vi "FPGA_brightfield_control.vi"() -> ()   [LabVIEW 2015]
uses:
  <vilib>/rvi/Emulation/niFpgaGetClockAttributes.vi
  <vilib>/rvi/Emulation/niFpgaSctlEmulationGetInTimedLoop.vi
  <vilib>/rvi/Emulation/niFpgaEmulationReportErrorSimple.vi
  <vilib>/rvi/Emulation/niFpgaProcessEmulError.vi
  <vilib>/rvi/eio/common/nirviEmuTemplateMethod_errors.vi
  <vilib>/rvi/Emulation/niFpgaCriticalErrorInLSC.vi
  <vilib>/eio/EIONode/EIONode.xnode
panel:
  in  "Period":u32
  in  "Triggers length (µs)":u32
  in  "stop":bool
  in  "Intensity":sgl
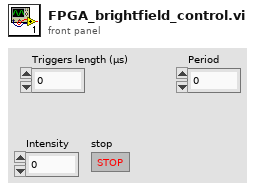
[diagram p1: front panel]
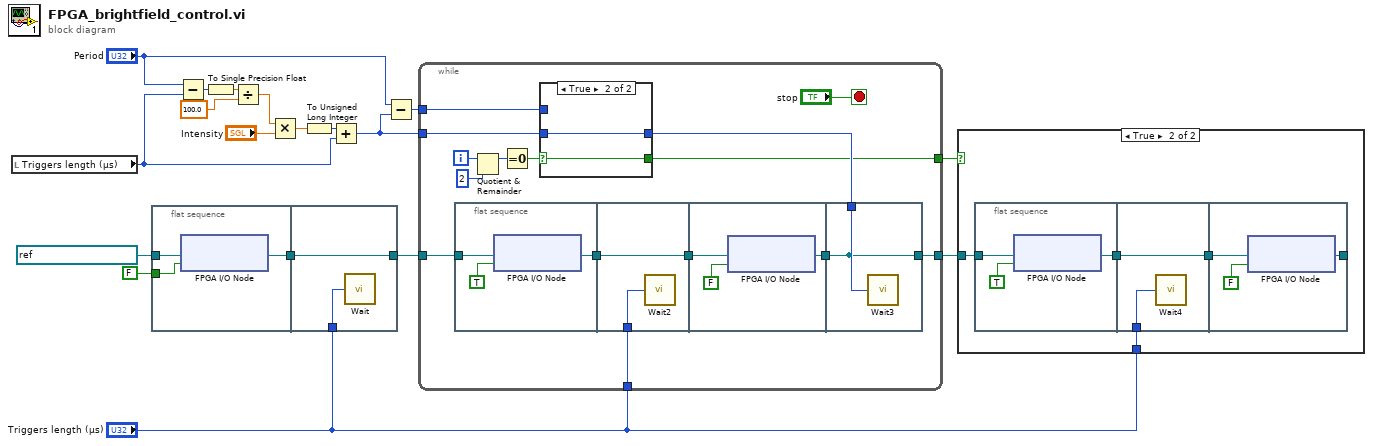
[diagram p0: block diagram]
diagram:
  n1 = local read "Triggers length (µs)"() -> (w6:u32)
  n2 = flat-sequence {
    tunnel: refnum<k21> "Connector0/DIO5" ("FPGA I/O In") -> [w21]
    tunnel: FALSE ("I/O Item") -> [w20]
    tunnel: [w19] -> w16
    tunnel: [w23] -> w15
    tunnel: w16 -> [w23]
    tunnel: "Triggers length (µs)" -> [w22]
    frame #0 {
      n3 = xnode "FPGA I/O Node"("I/O Item"=w20, "FPGA I/O In"=w21) -> ("FPGA I/O Out"=w19:refnum<k21>)
    }
    frame #1 {
      n4 = call "Wait"("Count(uSec)"=w22) -> ()  [unwired: 1 out]
    }
  }
  n5 = Subtract(x="Period", y=w6) -> (x-y=w5:u32)
  n6 = To Single Precision Float(number=w5) -> (single precision float=w1:sgl)
  n7 = Divide(x=w1, y=sgl 100.0) -> (x/y=w3:sgl)
  n8 = Multiply(x=w3, y="Intensity") -> (x*y=w8:sgl)
  n9 = To Unsigned Long Integer(number=w8) -> (unsigned 32bit integer=w9:u32)
  n10 = Add(x=w9, y=w6) -> (x+y=w7:u32)
  n11 = Subtract(x="Period", y=w7) -> (x-y=w13:u32)
  n12 = while {
    tunnel: w7 -> [w32]
    tunnel: w13 -> [w31]
    tunnel: w15 -> [w36]
    tunnel: [w27] -> w12
    tunnel: [w25] -> w11
    tunnel: "Triggers length (µs)" -> [w24]
    i -> [w26]
    stop <- "stop" stop-if-true
    n13 = flat-sequence {
      tunnel: [w44] -> w38
      tunnel: w36 -> [w43]
      tunnel: w38 -> [w47]
      tunnel: [w47] -> w37
      tunnel: w24 -> [w46]
      tunnel: w37 -> [w49]
      tunnel: [w48] -> w30
      tunnel: [w51] -> _
      tunnel: w30 -> [w51]
      tunnel: w29 -> [w52]
      tunnel: [w51] -> w25
      frame #0 {
        n14 = xnode "FPGA I/O Node"("I/O Item"=TRUE, "FPGA I/O In"=w43) -> ("FPGA I/O Out"=w44:refnum<k21>)
      }
      frame #1 {
        n15 = call "Wait2"("Count(uSec)"=w46) -> ()  [unwired: 1 out]
      }
      frame #2 {
        n16 = xnode "FPGA I/O Node"("I/O Item"=FALSE, "FPGA I/O In"=w49) -> ("FPGA I/O Out"=w48:refnum<k21>)
      }
      frame #3 {
        n17 = call "Wait3"("Count(uSec)"=w52) -> ()  [unwired: 1 out]
      }
    }
    n18 = Quotient & Remainder(x=w26, y=2) -> (x-y*floor(x/y)=w34:i32)  [unwired: 1 out]
    n19 = Equal To 0?(x=w34) -> (x = 0?=w33:bool)
    n20 = case shown="True" w33 {
      selector: w33 -> [w39 w41]
      tunnel: w32 -> [_ w42]
      tunnel: w31 -> [w40 _]
      tunnel: [w40 w42] -> w29
      tunnel: [w39 w41] -> w27
      frame False {
      }
      frame True {
      }
    }
  }
  n21 = case shown="True" w12 {
    tunnel: w11 -> [_ w54]
    tunnel: "Triggers length (µs)" -> [_ w53]
    frame False {
    }
    frame True {
      n22 = flat-sequence {
        tunnel: [w58] -> w56
        tunnel: w54 -> [w57]
        tunnel: w56 -> [w61]
        tunnel: [w61] -> w55
        tunnel: w53 -> [w60]
        tunnel: w55 -> [w63]
        tunnel: [w62] -> _
        frame #0 {
          n23 = xnode "FPGA I/O Node"("I/O Item"=TRUE, "FPGA I/O In"=w57) -> ("FPGA I/O Out"=w58:refnum<k21>)
        }
        frame #1 {
          n24 = call "Wait4"("Count(uSec)"=w60) -> ()  [unwired: 1 out]
        }
        frame #2 {
          n25 = xnode "FPGA I/O Node"("I/O Item"=FALSE, "FPGA I/O In"=w63) -> ("FPGA I/O Out"=w62:refnum<k21>)
        }
      }
    }
  }
